vi "Deformação e tensões.vi"(2 "Dados":T1, 3 "Resultados":dbl[][](array[numeric])) -> (0 "Derivada":cluster{"z":dbl[], "Array":dbl[]}[](array[cluster]), 1 "Gráfico":cluster{"z":dbl[], "Array":dbl[]}[](array[cluster]))   [LabVIEW 2018]
uses:
  <vilib>/Analysis/NI_AALPro.lvlib
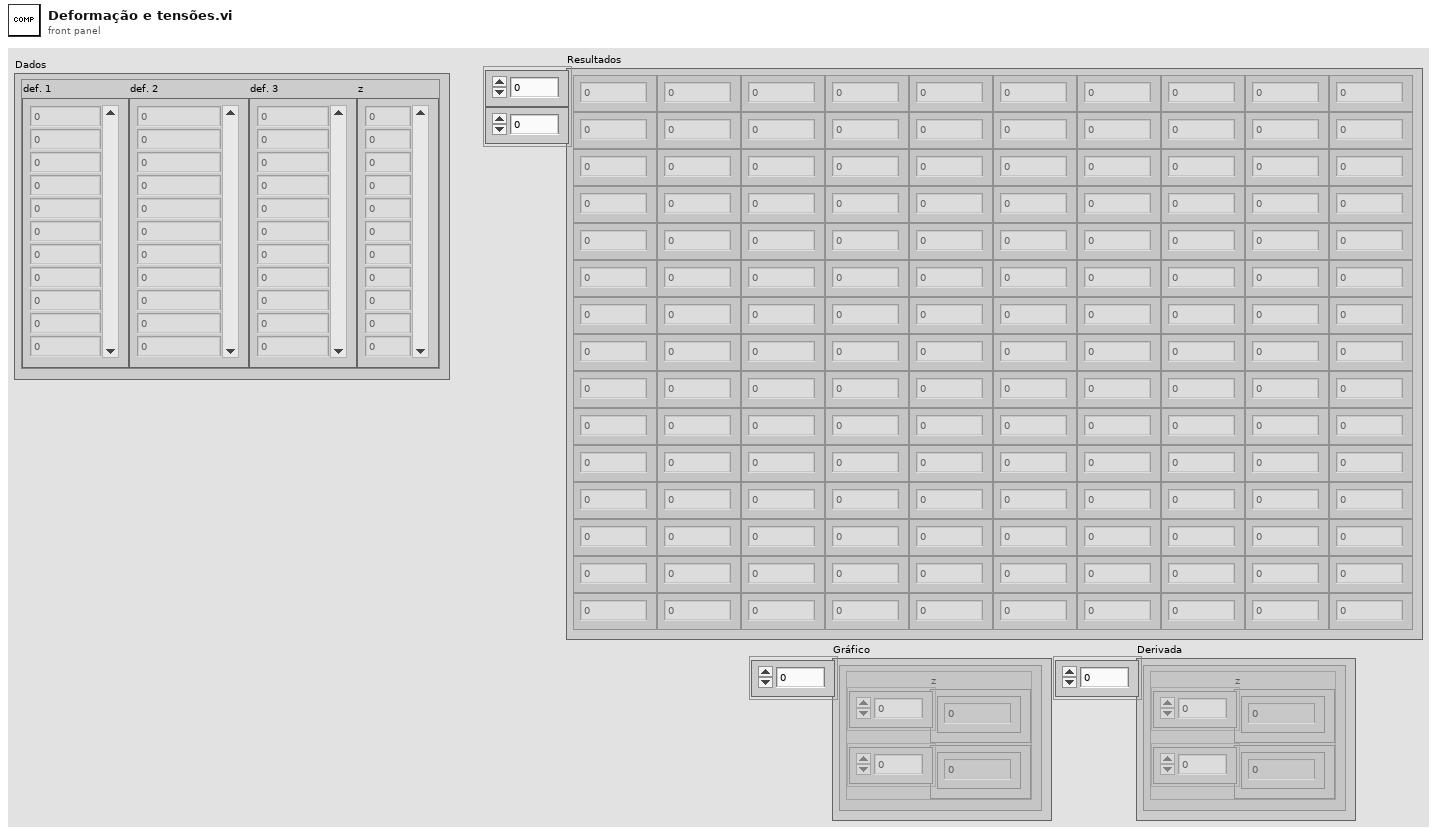
[diagram p1: front panel]
types:
  T1 = typedef "Deformações.ctl" = cluster{"def. 1 ":dbl[], "def. 2":dbl[], "def. 3":dbl[], "z":dbl[]}
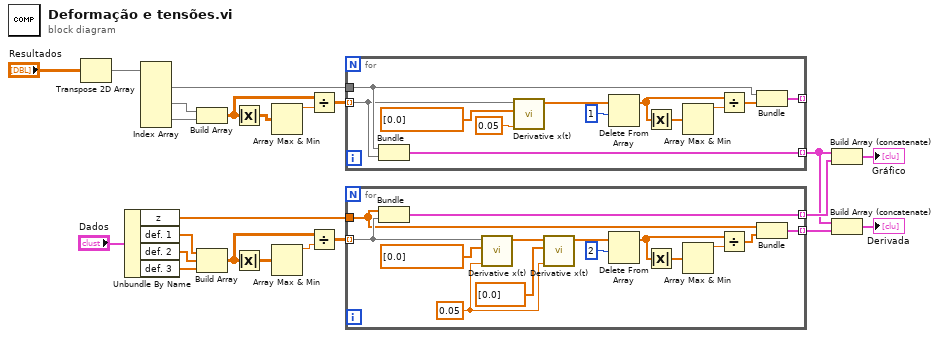
[diagram p0: block diagram]
diagram:
  n1 = Transpose 2D Array(2D array="Resultados") -> (transposed array=w13:dbl[][])
  n2 = Unbundle By Name("Dados") -> ("z"=w15:dbl[], "def. 1"=w22:dbl[], "def. 2"=w21:dbl[], "def. 3"=w20:dbl[])
  n3 = Index Array(array=w13) -> (element #1=w6:dbl[], element #2=w12:dbl[], element #3=w11:dbl[])  [unwired: 6 in]
  n4 = Build Array(w12, w11) -> (w8:dbl[][])
  n5 = Build Array(w22, w21, w20) -> (w17:dbl[][])
  n6 = Absolute Value(x=w8) -> (abs(x)=w9:dbl[][])
  n7 = Absolute Value(x=w17) -> (abs(x)=w19:dbl[][])
  n8 = Array Max & Min(array=w9) -> (max value=w10:dbl)  [unwired: 3 out]
  n9 = Array Max & Min(array=w19) -> (max value=w18:dbl)  [unwired: 3 out]
  n10 = Divide(x=w8, y=w10) -> (x/y=w7:dbl[][])
  n11 = Divide(x=w17, y=w18) -> (x/y=w16:dbl[][])
  n12 = for {
    tunnel: w7 -> [w24] mode=indexing
    tunnel: w6 -> [w26]
    tunnel: [w35] -> w1 mode=indexing
    tunnel: [w25] -> _ mode=indexing
    n13 = Bundle(w26, w24) -> (w35:cluster{dbl[], dbl[]})  [unwired: 1 in]
    n14 = call <vilib>:"Derivative x(t).vi"("dt"=0.05, "Initial Condition"=dbl[] [0.0], "X"=w24) -> ("dX/dt"=w28:dbl[])  [unwired: 7 in, 1 out]
    n15 = Delete From Array(array=w28, length=1) -> (array with subset deleted=w31:dbl[])  [unwired: 1 in, 1 out]
    n16 = Absolute Value(x=w31) -> (abs(x)=w30:dbl[])
    n17 = Array Max & Min(array=w30) -> (max value=w29:dbl)  [unwired: 3 out]
    n18 = Divide(x=w31, y=w29) -> (x/y=w27:dbl[])
    n19 = Bundle(w26, w27) -> (w25:cluster{dbl[], dbl[]})  [unwired: 1 in]
  }
  n20 = for {
    tunnel: w16 -> [w48] mode=indexing
    tunnel: w15 -> [w45]
    tunnel: [w49] -> w5 mode=indexing
    tunnel: [w44] -> w3 mode=indexing
    w47 = 0.05 ("dt")
    n21 = Bundle("z"=w45, w48) -> (w49:cluster{"z":dbl[], dbl[]})  [unwired: 1 in]
    n22 = call <vilib>:"Derivative x(t).vi"("dt"=w47, "Initial Condition"=dbl[] [0.0], "X"=w48) -> ("dX/dt"=w46:dbl[])  [unwired: 7 in, 1 out]
    n23 = call <vilib>:"Derivative x(t).vi"("dt"=w47, "Initial Condition"=dbl[] [0.0], "X"=w46) -> ("dX/dt"=w38:dbl[])  [unwired: 7 in, 1 out]
    n24 = Delete From Array(array=w38, length=2) -> (array with subset deleted=w37:dbl[])  [unwired: 1 in, 1 out]
    n25 = Absolute Value(x=w37) -> (abs(x)=w40:dbl[])
    n26 = Array Max & Min(array=w40) -> (max value=w41:dbl)  [unwired: 3 out]
    n27 = Divide(x=w37, y=w41) -> (x/y=w39:dbl[])
    n28 = Bundle("z"=w45, w39) -> (w44:cluster{"z":dbl[], dbl[]})  [unwired: 1 in]
  }
  n29 = Build Array (concatenate)(w1, w5) -> (→"Gráfico":cluster{"z":dbl[], dbl[]}[])
  n30 = Build Array (concatenate)(w1, w3) -> (→"Derivada":cluster{"z":dbl[], dbl[]}[])
